vi "Gobal for ROS.vi"() -> ()   [LabVIEW 2015, in "Biblioteka moduł map v3.lvlib" / "ROS.lvlib"]
uses:
  ROS.lvlib
panel:
  in  "String":string="GET / HTTP/1.1\nUpgrade: websocket\nConnection: Upgrade\nHost: 192.168.5.103:9090\nOrigin: http://192.168.5.101:9090\nSec-WebSocket-Key: pM4mFvl5nUXJXjxIa41LvQ==\nSec-WebSocket-Version: 13"
  in  "rosbridge port":u16=9090
  in  "rosbridge server IP":string="192.168.1.138"
  out "ROS read":T1
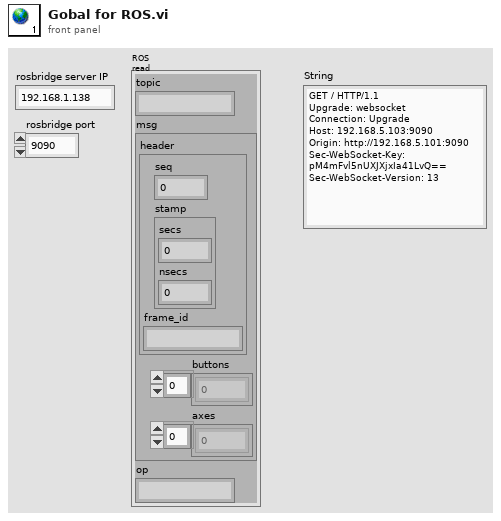
[diagram p1: front panel]
types:
  T1 = cluster{"topic":string, "msg":cluster{"header":cluster{"seq":u32, "stamp":cluster{"secs":u32, "nsecs":i32}, "frame_id":string}, "buttons":i32[], "axes":sgl[]}, "op":string}
diagram:
